vi "Store Session State.vi"(8 "error in (no error)":errorcluster, 11 "Session":refnum<class "Session.lvclass">) -> (0 "error out":errorcluster, 3 "Session dup":refnum<class "Session.lvclass">)   [LabVIEW 2013, in "MQTT Server.lvlib" / "StoredSessions.lvclass"]
uses:
  StoredSessions.lvclass
  <vilib>/LabVIEW Open Source Project/MQTT Connection/MQTT_Base/Session/Session.lvclass
  <vilib>/LabVIEW Open Source Project/MQTT Connection/MQTT_Base/Session/Session.lvclass/Session.ctl
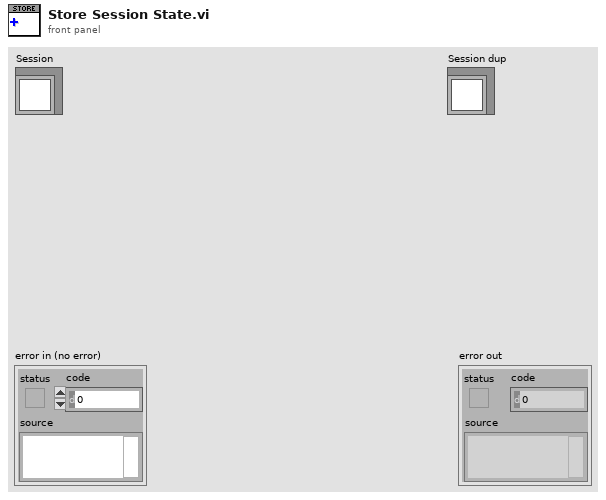
[diagram p1: front panel]
types:
  T1 = typedef "MQTT Base.lvlib/Session.lvclass/Session State -- cluster.ctl" = cluster{"CleanSession":bool, "Client ID":string, "Subscriptions":T2[], "Pending Transmissions":T4[], "Pending ACKs":T5[]}
  T2 = typedef "MQTT_Control_Packets.lvlib/SUBSCRIBE.lvclass/Topic Subscription -- cluster.ctl" = cluster{"Topic Filter":string, "QoS":T3}
  T3 = typedef "MQTT_Control_Packets.lvlib/ControlPacket.lvclass/QualityOfService -- enum.ctl" = enum16{"0 (At Most Once)", "1 (At Least Once)", "2 (Exactly Once)"}
  T4 = typedef "MQTT_Control_Packets.lvlib/ControlPacket.lvclass/Pending Transmission -- cluster.ctl" = cluster{"Message":refnum<class "ControlPacket.lvclass">, "QoS":T3, "Tx-Rx":bool}
  T5 = typedef "MQTT Base.lvlib/Session.lvclass/Pending ACKs -- cluster.ctl" = cluster{"Message":refnum<class "ControlPacket.lvclass">, "[ACK]":refnum<notifier>[], "Packet Identifier":u16}
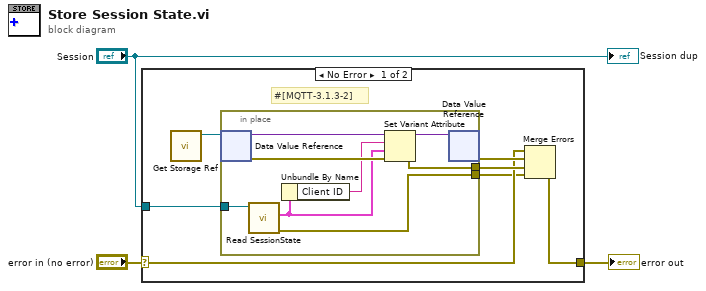
[diagram p0: block diagram]
diagram:
  n1 = case shown="No Error" "error in (no error)" {
    selector: "error in (no error)" -> [w6 w19]
    tunnel: [w5 w19] -> w2
    tunnel: "Session" -> [w9 _]
    frame No Error {
      # "#[MQTT-3.1.3-2]"
      n2 = call "Get Storage Ref.vi"() -> ("Storage"=w10:refnum<data-value>)  [unwired: 11 in]
      n3 = in-place {
        in-place-border: w9 -> [w14]
        in-place-border: [w16] -> w8
        in-place-border: [w13] -> w4
        n4 = in-place-dvr #1(w10) -> (w18:variant, w15:errorcluster)
        n5 = call <vilib>:"Read SessionState.vi"("Session in"=w14) -> ("error out"=w13:errorcluster, "Session State"=w12:T1)  [unwired: 8 in, 1 out]
        n6 = Unbundle By Name(w12) -> ("Client ID"=w11:string)
        n7 = Set Variant Attribute(Variant=w18, name=w11, value=w12, error in=w15) -> (Variant out=w17:variant, error out=w16:errorcluster)  [unwired: 1 out]
        n8 = in-place-dvr #1(w17) -> (w7:errorcluster)  [unwired: 1 out]
      }
      n9 = Merge Errors(w6, w7, w8, w4) -> (w5:errorcluster)
    }
    frame Error {
    }
  }
  "error out" <- w2
  "Session dup" <- "Session"
